vi "Create Sync Tool.vi"(7 "Reference Target Name":string, 8 "error in (no error)":errorcluster, 10 "Project Path":path) -> (0 "error out":errorcluster, 3 "CD Build Tools out":refnum<class "Project Sync Tools.lvclass">)   [LabVIEW 2019, in "Project Sync Tools.lvclass"]
uses:
  Project Sync Tools.lvclass
  Project Sync Tools.lvclass/Project Sync Tools.ctl
panel:
  out "Project Path out":path
  in  "error in (no error) 2":errorcluster
  out "error out 2":errorcluster
  out "Build Specification Names 2":string[](array[string])
  in  "Project Path in":path
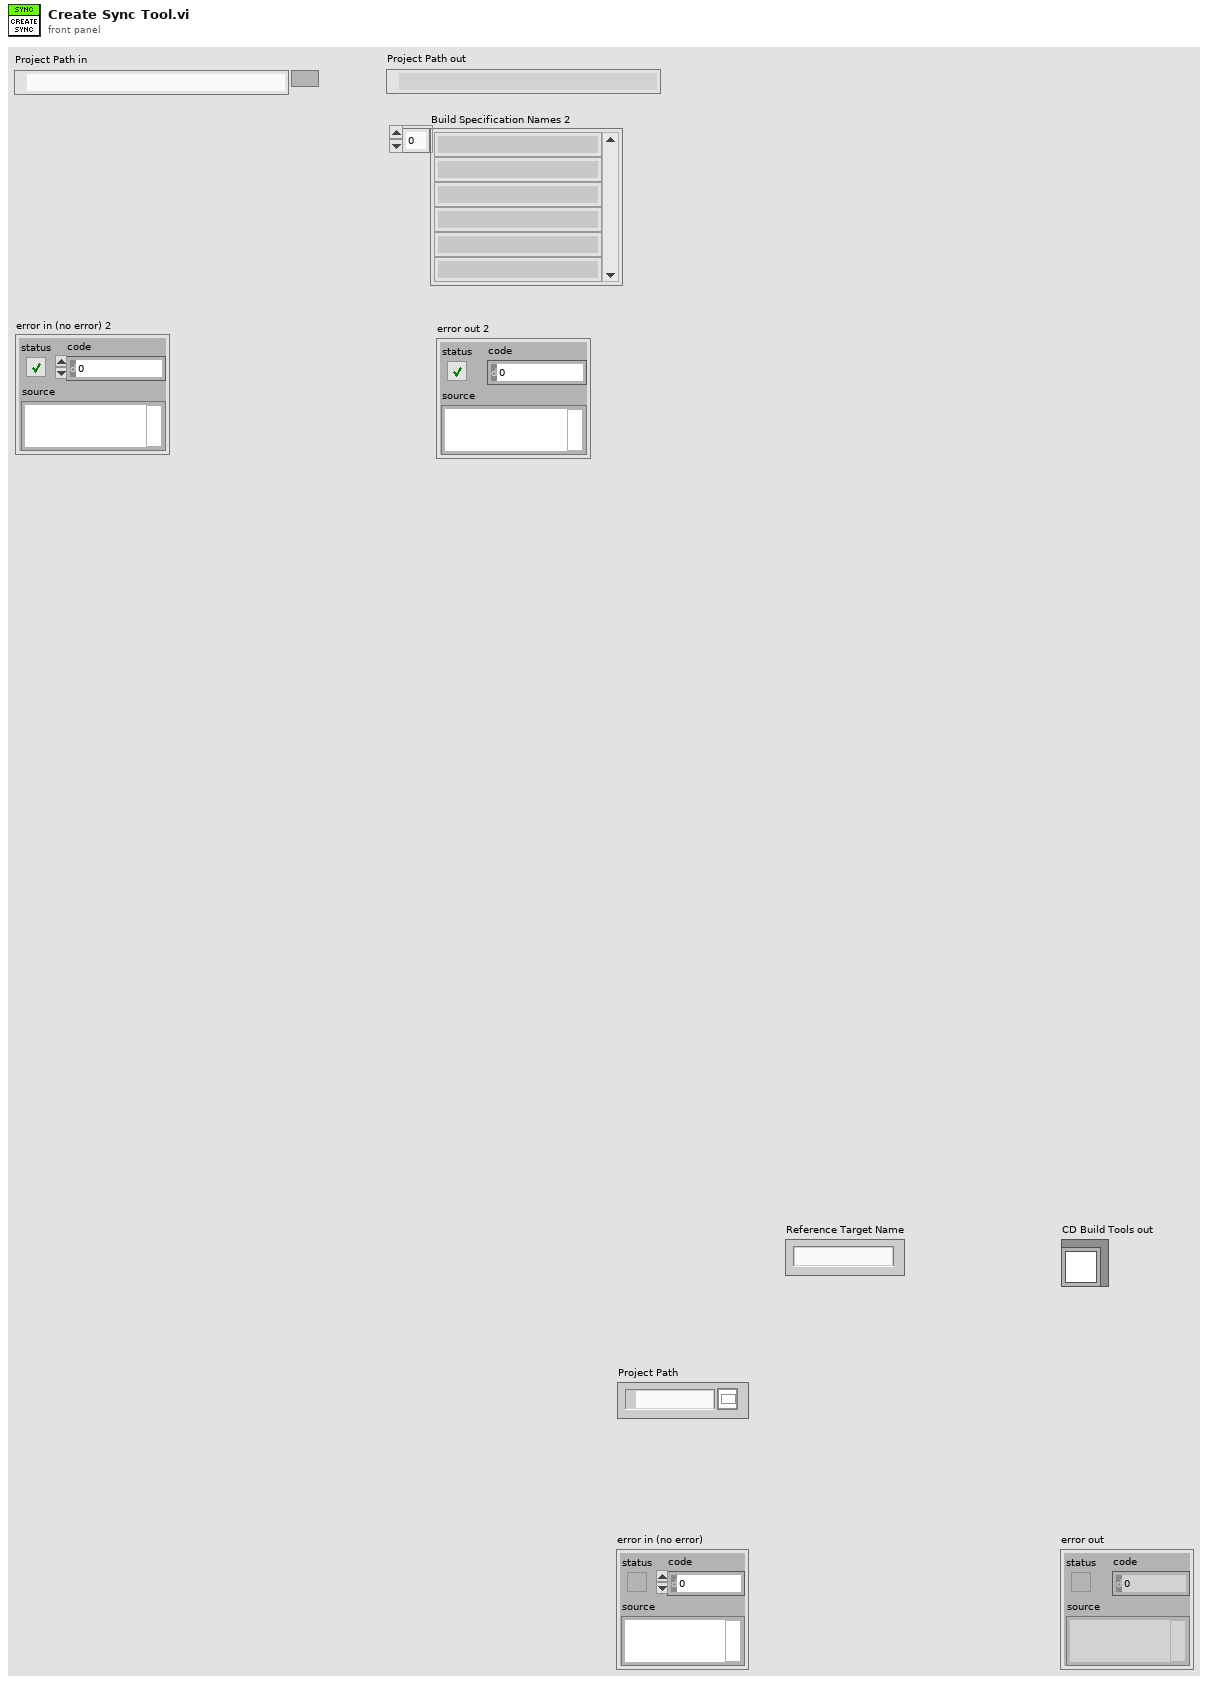
[diagram p1: front panel]
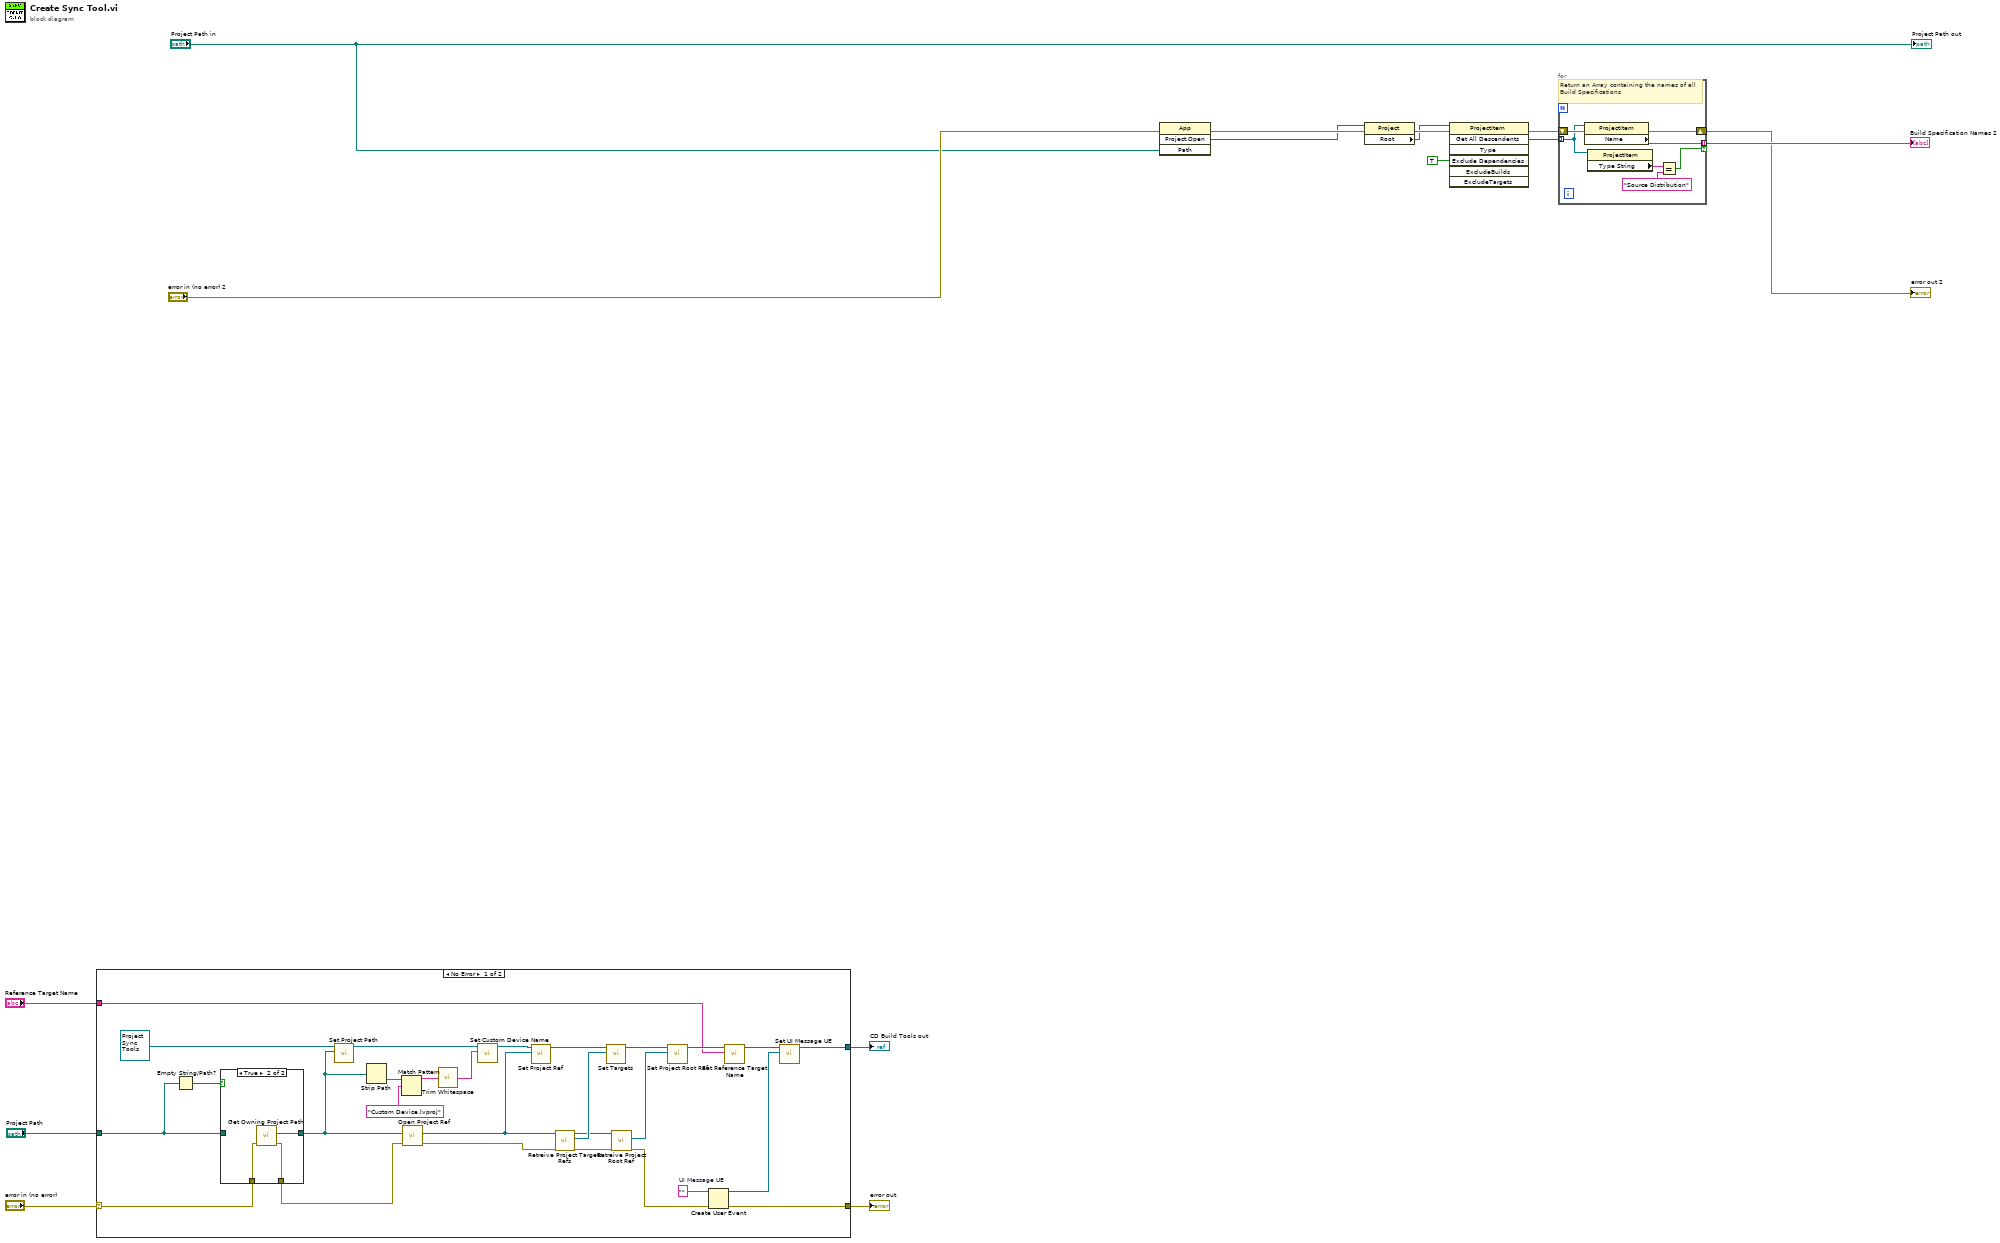
[diagram p0: block diagram]
diagram:
  n1 = case shown="No Error" "error in (no error)" {
    selector: "error in (no error)" -> [w41 w50]
    tunnel: [w26 w50] -> w15
    tunnel: [w24 _] -> w14
    tunnel: "Project Path" -> [w42 _]
    tunnel: "Reference Target Name" -> [w30 _]
    frame No Error {
      w29 = ""  # UI Message UE
      n2 = Empty String/Path?(string/path=w42) -> (empty?=w43:bool)
      n3 = case shown="True" w43 {
        tunnel: [w46 w48] -> w18
        tunnel: w42 -> [w46 _]
        tunnel: w41 -> [w45 w49]
        tunnel: [w45 w47] -> w40
        frame False {
        }
        frame True {
          n4 = call "Get Owning Project Path.vi"("error in (no error)"=w49) -> ("error out"=w47:errorcluster, "Path"=w48:path)  [unwired: 9 in]
        }
      }
      n5 = call "Set Project Path.vi"("Project Path"=w18, "CD Build Tools in"=refnum<class "Project Sync Tools.lvclass"> refnum ("CD Build Tools out")) -> ("CD Build Tools out"=w23:refnum<class "Project Sync Tools.lvclass">)  [unwired: 9 in]
      n6 = Strip Path(path=w18) -> (name=w21:string)  [unwired: 1 out]
      n7 = Match Pattern(string=w21, regular expression="Custom Device.lvproj") -> (before substring=w20:string)  [unwired: 1 in, 3 out]
      n8 = call "Open Project Ref.vi"("error in (no error)"=w40, "Project Path"=w18) -> ("error out"=w32:errorcluster, "Project Ref out"=w38:refnum<vi>)  [unwired: 8 in]
      n9 = call <vilib>:"Trim Whitespace.vi"("string"=w20) -> ("trimmed string"=w17:string)  [unwired: 1 in]
      n10 = call "Set Custom Device Name.vi"("Custom Device Name"=w17, "Project Sync Tools in"=w23) -> ("Project Sync Tools out"=w22:refnum<class "Project Sync Tools.lvclass">)  [unwired: 8 in, 1 out]
      n11 = call "Set Project Ref.vi"("Project Ref"=w38, "CD Build Tools in"=w22) -> ("CD Build Tools out"=w37:refnum<class "Project Sync Tools.lvclass">)  [unwired: 9 in]
      n12 = call "Retreive Project Targets Refs.vi"("error in (no error)"=w32, "Project in"=w38) -> ("error out"=w35:errorcluster, "Targets"=w36:refnum<vi>[], "Project out"=w34:refnum<vi>)  [unwired: 7 in]
      n13 = call "Set Targets.vi"("Targets"=w36, "Project Sync Tools in"=w37) -> ("Project Sync Tools out"=w33:refnum<class "Project Sync Tools.lvclass">)  [unwired: 9 in]
      n14 = call "Retreive Project Root Ref.vi"("error in (no error)"=w35, "Project in"=w34) -> ("error out"=w27:errorcluster, "Project Root out"=w39:refnum<vi>)  [unwired: 7 in, 1 out]
      n15 = call "Set Project Root Ref.vi"("Project Root Ref"=w39, "CD Build Tools in"=w33) -> ("CD Build Tools out"=w31:refnum<class "Project Sync Tools.lvclass">)  [unwired: 9 in]
      n16 = Create User Event(user event datatype=w29, error in=w27) -> (user event=w25:refnum<user-event>, error out=w26:errorcluster)
      n17 = call "Set Reference Target Name.vi"("Reference Target Name"=w30, "Project Sync Tools in"=w31) -> ("Project Sync Tools out"=w28:refnum<class "Project Sync Tools.lvclass">)  [unwired: 9 in]
      n18 = call "Set UI Message UE.vi"("UI Message UE"=w25, "Project Sync Tools in"=w28) -> ("Project Sync Tools out"=w24:refnum<class "Project Sync Tools.lvclass">)  [unwired: 9 in]
    }
    frame Error {
    }
  }
  "error out" <- w15
  "CD Build Tools out" <- w14
  n19 = invoke class="App" method="Project.Open"(error in="error in (no error) 2", "Path"="Project Path in") -> (error out=w10:errorcluster, "Project:Open"=w9:refnum<vi>)  [unwired: 2 in, 2 out]
  n20 = property class="Project"(reference=w9, error in=w10) -> (error out=w12:errorcluster, "Root"=w11:refnum<vi>)  [unwired: 1 out]
  n21 = invoke class="ProjectItem" method="Get All Descendents"(reference=w11, error in=w12, "Exclude Dependencies"=TRUE ("ExcludeDependencies")) -> (error out=w7:errorcluster, "All Descendents"=w8:refnum<vi>[])  [unwired: 4 in, 5 out]
  n22 = for {
    tunnel: w8 -> [w54] mode=indexing
    tunnel: [w57] -> w6 mode=indexing if=w51
    shift-right: [w55] -> w4
    shift-left: w7 -> [w56]
    # "Return an Array containing the names of all Build Specifications"
    n23 = property class="ProjectItem"(reference=w54, error in=w56) -> (error out=w55:errorcluster, "Name"=w57:string)  [unwired: 1 out]
    n24 = property class="ProjectItem"(reference=w54) -> ("Type String"=w53:string)  [unwired: 1 in, 2 out]
    n25 = Equal?(x=w53, y="Source Distribution") -> (x = y?=w51:bool)
  }
  "Build Specification Names 2" <- w6
  "error out 2" <- w4
  "Project Path out" <- "Project Path in"
